vi "Close.vi"(8 "error in (no error)":errorcluster, 11 "Data in":refnum<class "FPGA-Bus.lvclass">) -> (0 "error out":errorcluster, 3 "Data out":refnum<class "FPGA-Bus.lvclass">)   [LabVIEW 2021, in "FPGA-Bus.lvclass"]
uses:
  FPGA-Bus.lvclass
  <vilib>/TSA/Omni-Bus/Omni-Bus/Bus Access/Bus_Access.lvclass
  FPGA-Bus.lvclass/FPGA-Bus.ctl
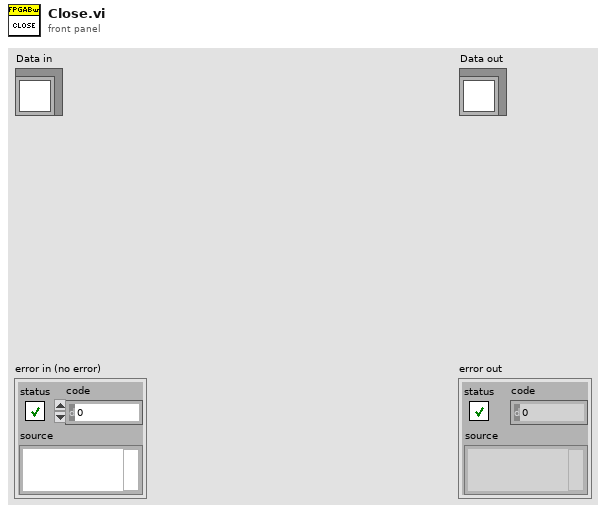
[diagram p1: front panel]
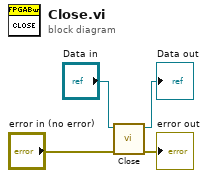
[diagram p0: block diagram]
diagram:
  n1 = call-parent "Close.vi"("error in (no error)"="error in (no error)", "Data in"="Data in") -> ("error out"=→"error out":errorcluster, "Data out"=→"Data out":refnum<class "FPGA-Bus.lvclass">)  [unwired: 8 in]
